vi "Do.vi"(8 "error in":errorcluster, 10 "Actor in":refnum<class "Actor.lvclass">, 11 "Change Speaker Vparams":refnum<class "Change Speaker Vparams MSG.lvclass">) -> (0 "error out":errorcluster, 2 "Actor out":refnum<class "Actor.lvclass">)   [LabVIEW 2014, in "ePAS Library.lvlib" / "Change Speaker Vparams MSG.lvclass"]
doc: "(<B>Filename</B>: Actor Framework.lvlib:Message.lvclass:Do.vi)\n\nDefines what a message does when it is received by an actor. Generally, a message instructs an actor to invoke one of its methods. By default, this method does nothing. A child class must override it to define behavior. Create a child class by using the Actor Framework Message Maker dialog box."
uses:
  Change Speaker Vparams MSG.lvclass
  <vilib>/ActorFramework/Actor/Actor.lvclass
  Change Speaker Vparams MSG.lvclass/Change Speaker Vparams MSG.ctl
  Instr Actor.lvclass
  PAS/Commands/Change Speaker Vparams/Change Speaker Vparams.lvclass
  PAS/Commands/Change Speaker Vparams/Change Speaker Vparams.lvclass/Change Speaker Vparams.ctl
  Controller/Messages/Update CVT/Update CVT Data.lvclass
  Controller/Messages/Update CVT/Update CVT Data.lvclass/Update CVT Data.ctl
  Controller/Messages/Update CVT/Write tag.vi
  Controller/Messages/Update CVT/Write Data.vi
  Controller/Messages/Update CVT/Write Group.vi
  PAS/Commands/Change Speaker Vparams/Write Voffset.vi
  PAS/Commands/Change Speaker Vparams/Write Vrange.vi
  reusable/Command/Command.lvclass
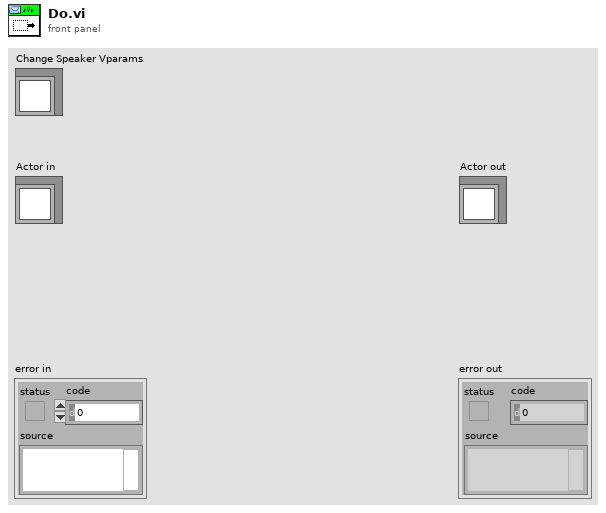
[diagram p1: front panel]
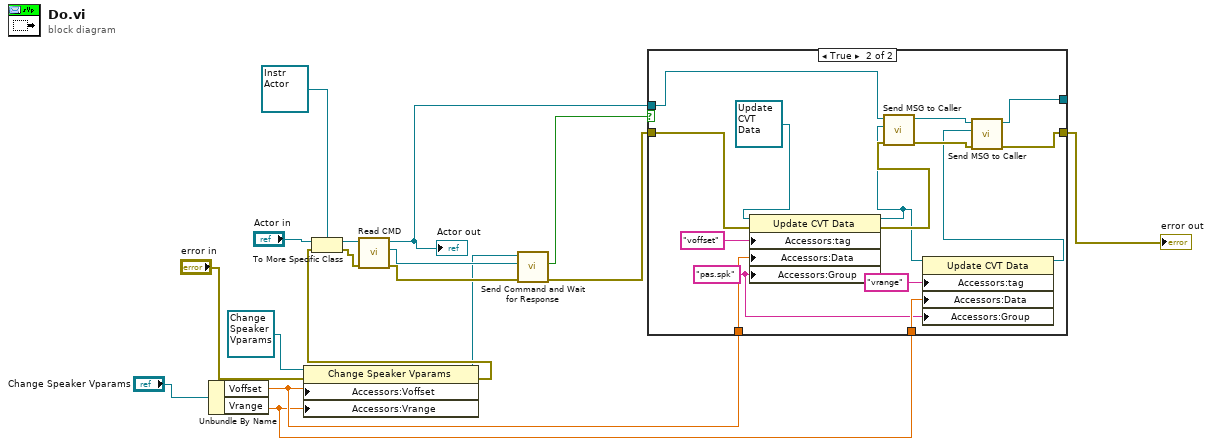
[diagram p0: block diagram]
diagram:
  n1 = Unbundle By Name("Change Speaker Vparams") -> ("Voffset"=w2:dbl, "Vrange"=w1:dbl)
  n2 = property class="Change Speaker Vparams"(reference=refnum<class "Change Speaker Vparams.lvclass"> refnum ("Change Speaker Vparams"), error in="error in", "Accessors:Voffset"=w2, "Accessors:Vrange"=w1) -> (reference out=w7:refnum<class "Change Speaker Vparams.lvclass">, error out=w10:errorcluster)
  n3 = To More Specific Class(target class=refnum<class "Instr Actor.lvclass"> refnum ("Instrument Lib:Instr"), reference="Actor in", error in=w10) -> (specific class reference=w16:refnum<class "Instr Actor.lvclass">, error out=w15:errorcluster)
  n4 = call "Read CMD.vi"("error in (no error)"=w15, "Instr Actor in"=w16) -> ("error out"=w9:errorcluster, "CMD"=w8:refnum<queue>, "Instr Actor out"=w4:refnum<class "Instr Actor.lvclass">)  [unwired: 7 in]
  "Actor out" <- w4
  n5 = call "Send Command and Wait for Response.vi"("error in"=w9, "cmd queue"=w8, "CMD in"=w7) -> ("error out"=w5:errorcluster, "cmd good?"=w6:bool)  [unwired: 6 in, 1 out]
  n6 = case shown="True" w6 {
    tunnel: w4 -> [w19 w31]
    tunnel: [w19 w28] -> _
    tunnel: w5 -> [w18 w33]
    tunnel: [w18 w27] -> w3
    tunnel: w2 -> [_ w25]
    tunnel: w1 -> [_ w24]
    frame False {
    }
    frame True {
      w20 = "pas.spk" ("Group")
      n7 = property class="Update CVT Data"(reference=refnum<class "Update CVT Data.lvclass"> refnum ("Controller.lvlib:Update CVT Data"), error in=w33, "Accessors:tag"="voffset" ("Key"), "Accessors:Data"=w25, "Accessors:Group"=w20) -> (reference out=w26:refnum<class "Update CVT Data.lvclass">, error out=w32:errorcluster)
      n8 = call "Send MSG to Caller.vi"("error in"=w32, "Message"=w26, "Instr in"=w31) -> ("error out"=w29:errorcluster, "Instr out"=w30:refnum<class "Instr Actor.lvclass">)  [unwired: 7 in]
      n9 = property class="Update CVT Data"(reference=w26, "Accessors:tag"="vrange" ("Key"), "Accessors:Data"=w24, "Accessors:Group"=w20) -> (reference out=w22:refnum<class "Update CVT Data.lvclass">)  [unwired: 1 in, 1 out]
      n10 = call "Send MSG to Caller.vi"("error in"=w29, "Message"=w22, "Instr in"=w30) -> ("error out"=w27:errorcluster, "Instr out"=w28:refnum<class "Instr Actor.lvclass">)  [unwired: 7 in]
    }
  }
  "error out" <- w3
